vi "Instrument Manager.vi"(6 "Source":string="$.Instruments", 7 "Operation":T1(ring), 8 "error in":errorcluster, 11 "Instrument Identifier":string) -> (0 "error out":errorcluster)   [LabVIEW 2025, in "Instrument Manager AE.lvlib"]
uses:
  Instrument Manager AE.lvlib
  Interfaces/IInstrument/IInstrument.lvclass
  Config from JSON/Config from JSON.lvclass
  7ea29ae2-d732-4de8-820a-e720c47613e5.vi
  7ea29ae2-d732-4de8-820a-e720c47613e5.vi/a4169a97-72fc-4003-a778-603cf20cafa0.vi
  <vilib>/Utility/error.llb/Trim Whitespace.vi
  <vilib>/JDP Science/JSONtext/Find Item.vi
  <vilib>/Utility/error.llb/Trim Whitespace One-Sided.vi
  <vilib>/JDP Science/JSONtext/Next JSON Value.vi
  <vilib>/JDP Science/JSONtext/String Subset.vi
  <vilib>/JDP Science/JSONtext/Parsing/Advance past next JSON Value (inlined COPY).vi
  <vilib>/JDP Science/JSONtext/Parsing/Advance past whitespace.vi
  <vilib>/JDP Science/JSONtext/Parsing/Advance past String.vi
  <vilib>/JDP Science/JSONtext/Parsing/Advance past Number.vi
  <vilib>/JDP Science/JSONtext/Parsing/Advance past Line Ending.vi
  <vilib>/JDP Science/JSONtext/Parsing/Parse Full Path or Item Name.vi
  <vilib>/JDP Science/JSONtext/Parsing/Advance past Array.vi
  <vilib>/JDP Science/JSONtext/Parsing/Advance past Object.vi
  <vilib>/JDP Science/JSONtext/support/Error Cluster From Code.vi
  <vilib>/JDP Science/JSONtext/Offset/Find Item Locations by Path.vi
  <vilib>/JDP Science/JSONtext/JSON text to Variant.vi
  Common-LabVIEW-Helpers/Source/errors/-8301 Item not found in JSON--error.vi
  Common-LabVIEW-Helpers/Source/errors/-8300 JSON empty--error.vi
  <vilib>/JDP Science/JSONtext/LVClass Serializer/JSONtext LVClass Serializer.lvclass
panel:
  out "IInstrument":refnum<class "IInstrument.lvclass">
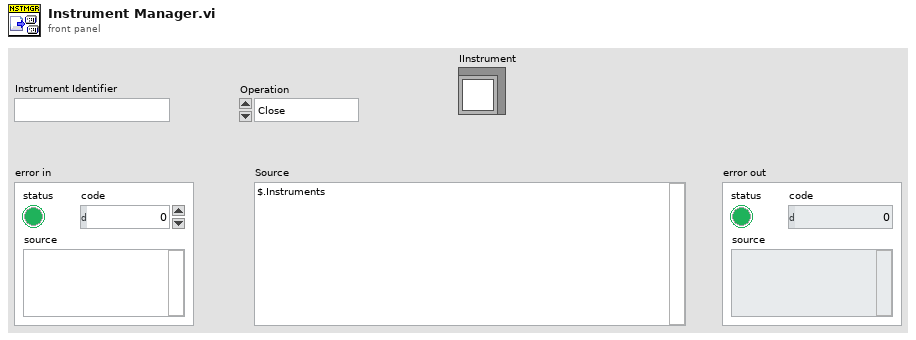
[diagram p1: front panel]
types:
  T1 = enum16{"Close", "Close Instrument", "Load Instruments", "Get Instrument"}
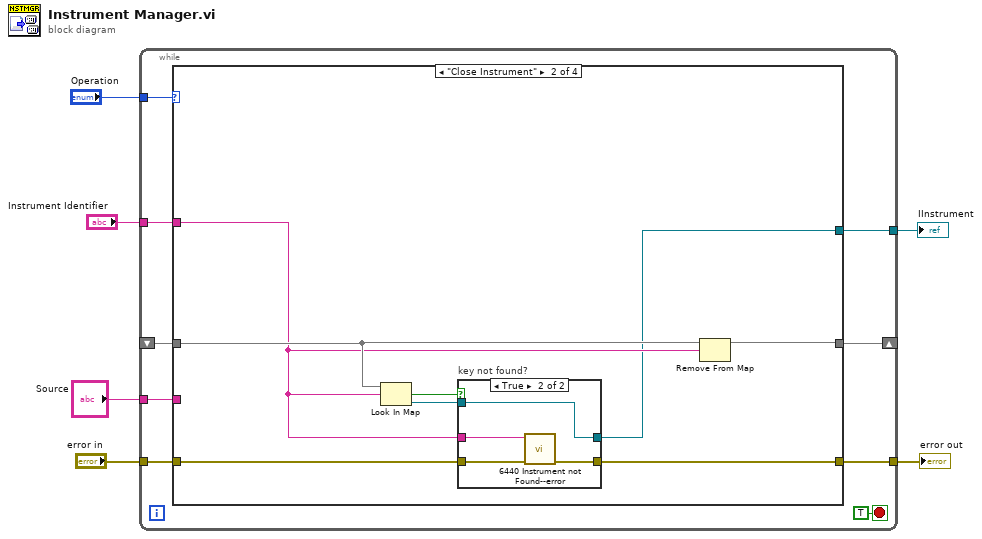
[diagram p0: block diagram]
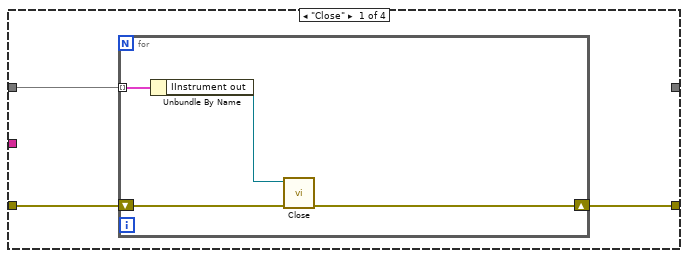
[diagram p2: hidden frame]
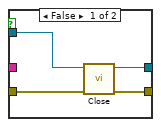
[diagram p3: hidden frame]
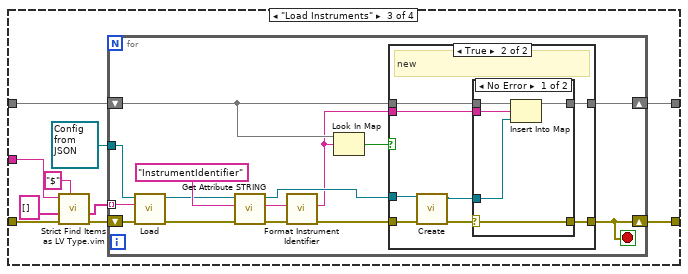
[diagram p4: hidden frame]
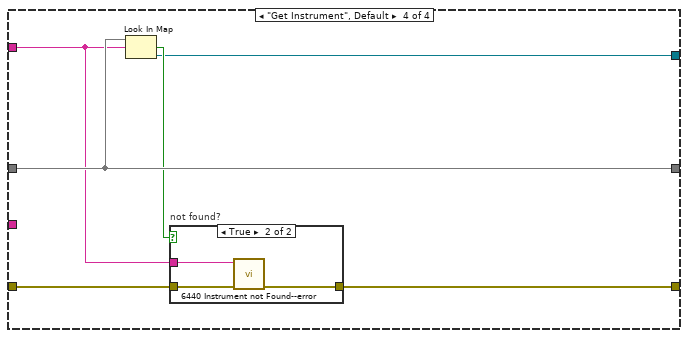
[diagram p7: hidden frame]
diagram:
  n1 = while {
    tunnel: "Operation" -> [w15]
    tunnel: "Source" -> [w14]
    shift-right: [w12] -> _
    shift-left: _ -> [w13]
    tunnel: "Instrument Identifier" -> [w11]
    tunnel: "error in" -> [w10]
    tunnel: [w9] -> w2
    tunnel: [w8] -> w1
    stop <- TRUE stop-if-true
    n2 = case shown="\"Close Instrument\"" w15 {
      tunnel: w14 -> [_ _ w47 _]
      tunnel: w13 -> [w18 w26 w44 w85]
      tunnel: [_ w24 w43 w85] -> w12
      tunnel: w11 -> [_ w25 _ w82]
      tunnel: w10 -> [w17 w28 w41 w84]
      tunnel: [w16 w27 w40 w83] -> w9
      tunnel: [_ w23 _ w80] -> w8
      frame "Close" {
        n3 = for {
          tunnel: w18 -> [w22] mode=indexing
          shift-right: [w19] -> w16
          shift-left: w17 -> [w20]
          n4 = Unbundle By Name(w22) -> ("IInstrument out"=w21:refnum<class "IInstrument.lvclass">)
          n5 = call-dynamic "Close.vi"("error in"=w20, "IClose in"=w21) -> ("error out"=w19:errorcluster)  [unwired: 8 in, 1 out]
        }
      }
      frame "Close Instrument" {
        n6 = Look In Map(map=w26, key=w25) -> (key not found?=w30:bool, value=w29:refnum<class "IInstrument.lvclass">)  [unwired: 1 in]
        n7 = case "key not found?" shown="True" w30 {
          tunnel: w29 -> [w32 w35]
          tunnel: w28 -> [w34 w38]
          tunnel: [w33 w37] -> w27
          tunnel: w25 -> [_ w36]
          tunnel: [w31 w35] -> w23
          frame False {
            n8 = call-dynamic "Close.vi"("error in"=w34, "IClose in"=w32) -> ("error out"=w33:errorcluster, "IClose out"=w31:refnum<class "IInstrument.lvclass">)  [unwired: 8 in]
          }
          frame True {
            n9 = call "6440 Instrument not Found--error.vi"("error in"=w38, "Argument"=w36) -> ("error out"=w37:errorcluster)  [unwired: 8 in, 1 out]
          }
        }
        n10 = Remove From Map(10:w25, 11:w26) -> (3:w24:map{string, refnum<class "IInstrument.lvclass">})  [unwired: 2 out]
      }
      frame "Load Instruments" {
        n11 = call "Strict Find Items as LV Type.vim"("$Path or Item Name"="$", "error in"=w41, "Data Type and Default Value"=string[] [], "<JSON>"=w47) -> ("error out"=w45:errorcluster, "Data out"=w42:string[])  [unwired: 5 in, 1 out]
        n12 = for {
          tunnel: w42 -> [w61] mode=indexing
          tunnel: refnum<class "Config from JSON.lvclass"> refnum ("Config From JSON in") -> [w60]
          shift-right: [w50] -> w43
          shift-left: w44 -> [w52]
          shift-right: [w49] -> w40
          shift-left: w45 -> [w57]
          stop <- w49 stop-if-true
          n13 = call-dynamic "Load.vi"("error in"=w57, "Source"=w61, "Config From JSON in"=w60) -> ("error out"=w58:errorcluster, "Config From JSON out"=w59:refnum<class "Config from JSON.lvclass">)  [unwired: 7 in]
          n14 = call-dynamic "Get Attribute STRING.vi"("error in"=w58, "Attribute"="InstrumentIdentifier" ("$Path or Item Name"), "ConfigFromJSON in"=w59) -> ("error out"=w54:errorcluster, "Value"=w55:string, "ConfigFromJSON out"=w56:refnum<class "Config from JSON.lvclass">)  [unwired: 6 in]
          n15 = call "Format Instrument Identifier.vi"("Identifier"=w55) -> ("Formatted Identifier"=w51:string)  [unwired: 10 in]
          n16 = Look In Map(map=w52, key=w51) -> (key not found?=w53:bool)  [unwired: 1 in, 1 out]
          n17 = case shown="True" w53 {
            tunnel: w56 -> [_ w71]
            tunnel: w54 -> [w64 w72]
            tunnel: w52 -> [w63 w69]
            tunnel: w51 -> [_ w68]
            tunnel: [w63 w67] -> w50
            tunnel: [w64 w65] -> w49
            frame False {
              # "not new"
            }
            frame True {
              # "new"
              n18 = call "Create.vi"("error in"=w72, "IConfiguration"=w71) -> ("error out"=w70:errorcluster, "IInstrument out"=w66:refnum<class "IInstrument.lvclass">)  [unwired: 8 in]
              n19 = case shown="No Error" w70 {
                selector: w70 -> [w73 w78]
                tunnel: w69 -> [w77 w79]
                tunnel: w68 -> [w76 _]
                tunnel: [w75 w79] -> w67
                tunnel: w66 -> [w74 _]
                tunnel: [w73 w78] -> w65
                frame No Error {
                  n20 = Insert Into Map(map in=w77, key=w76, value=w74) -> (map out=w75:map{string, refnum<class "IInstrument.lvclass">})  [unwired: 2 out]
                }
                frame Error {
                }
              }
            }
          }
        }
      }
      frame "Get Instrument", Default {
        n21 = Look In Map(map=w85, key=w82) -> (key not found?=w81:bool, value=w80:refnum<class "IInstrument.lvclass">)  [unwired: 1 in]
        n22 = case "not found?" shown="True" w81 {
          tunnel: w84 -> [w86 w89]
          tunnel: [w86 w88] -> w83
          tunnel: w82 -> [_ w87]
          frame False {
          }
          frame True {
            n23 = call "6440 Instrument not Found--error.vi"("error in"=w89, "Argument"=w87) -> ("error out"=w88:errorcluster)  [unwired: 8 in, 1 out]
          }
        }
      }
    }
  }
  "error out" <- w2
  "IInstrument" <- w1
